vi "Create Tick Object.vi"(6 "Label Cluster In":T2, 8 "error in (no error)":errorcluster, 9 "Actual Range In":T1, 10 "3D Plot.lvclass in":refnum<class "3D Plot.lvclass">, 11 "Axis Object In":refnum<vi>) -> (0 "error out":errorcluster, 1 "Actual Range Out":T1, 2 "3D Plot.lvclass out":refnum<class "3D Plot.lvclass">, 3 "Axis Object Out":refnum<vi>, 4 "Label Cluster Out":T2)   [LabVIEW 2020, in "3D Plot.lvclass"]
uses:
  <vilib>/Math Plots/3D Math Plots/3D Plot/3D Plot/3D Plot.lvclass
  <vilib>/Math Plots/3D Math Plots/3D Plot/3D Plot/Typedef/Tick Array Cluster.ctl
  <vilib>/Math Plots/3D Math Plots/3D Plot/3D Plot/Typedef/Tick Array.ctl
  <vilib>/Math Plots/3D Math Plots/3D Plot/3D Plot/Typedef/Range Clusters.ctl
  <vilib>/Math Plots/3D Math Plots/3D Plot/3D Plot/3D Plot.lvclass/3D Plot.ctl
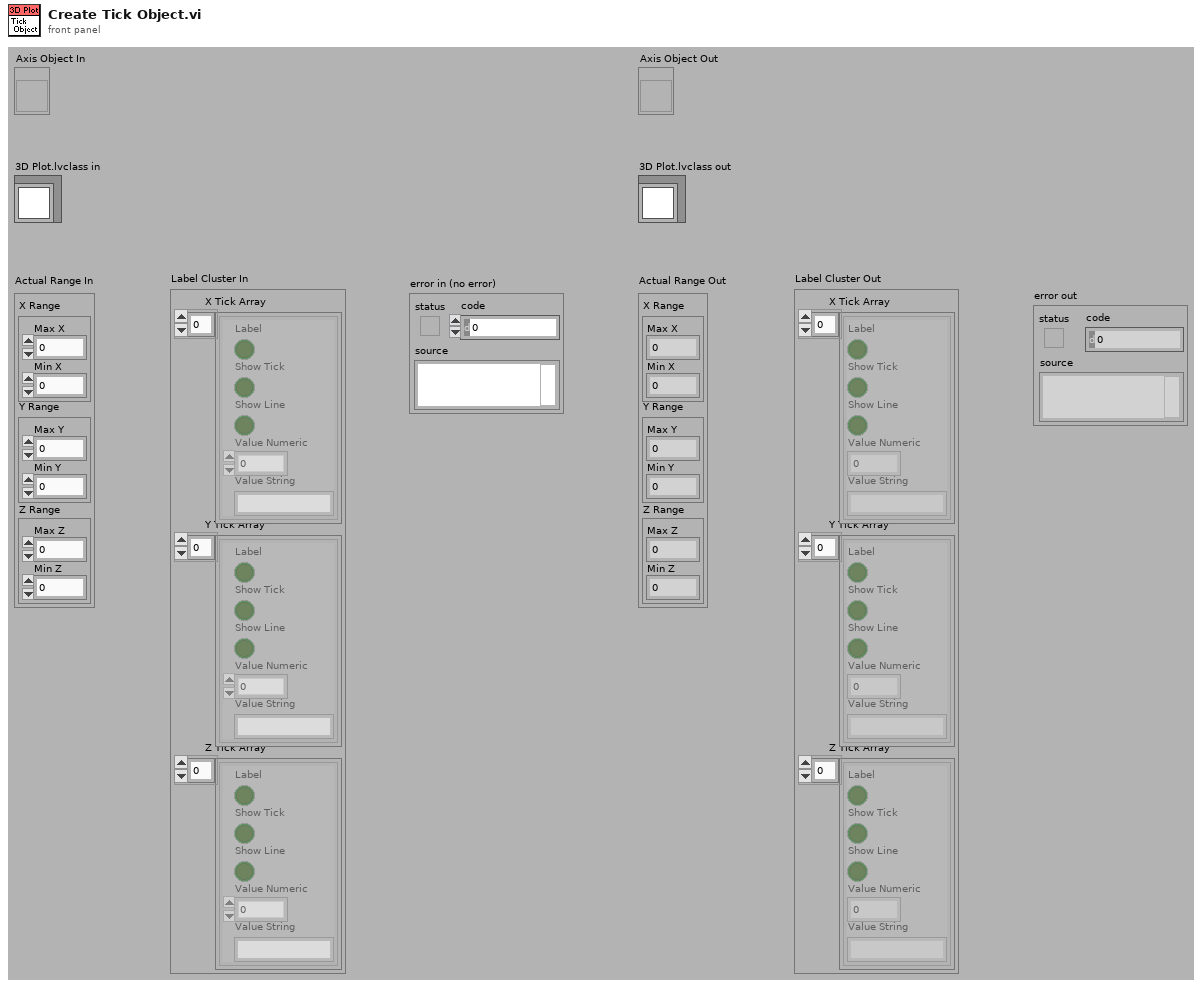
[diagram p1: front panel]
types:
  T1 = typedef "3D Plot.lvclass/Range Clusters.ctl" = cluster{"X Range":cluster{"Max X":sgl, "Min X":sgl}, "Y Range":cluster{"Max Y":sgl, "Min Y":sgl}, "Z Range":cluster{"Max Z":sgl, "Min Z":sgl}}
  T2 = typedef "3D Plot.lvclass/Tick Array Cluster.ctl" = cluster{"X Tick Array":T3, "Y Tick Array":T3, "Z Tick Array":T3}
  T3 = typedef "3D Plot.lvclass/Tick Array.ctl" = cluster{"Label":bool, "Show Tick":bool, "Show Line":bool, "Value Numeric":sgl, "Value String":string}[]
  T4 = cluster{"Draw Grid Plane X-Y":bool, "Draw Grid Plane Y-Z":bool, "Draw Grid Plane X-Z":bool}
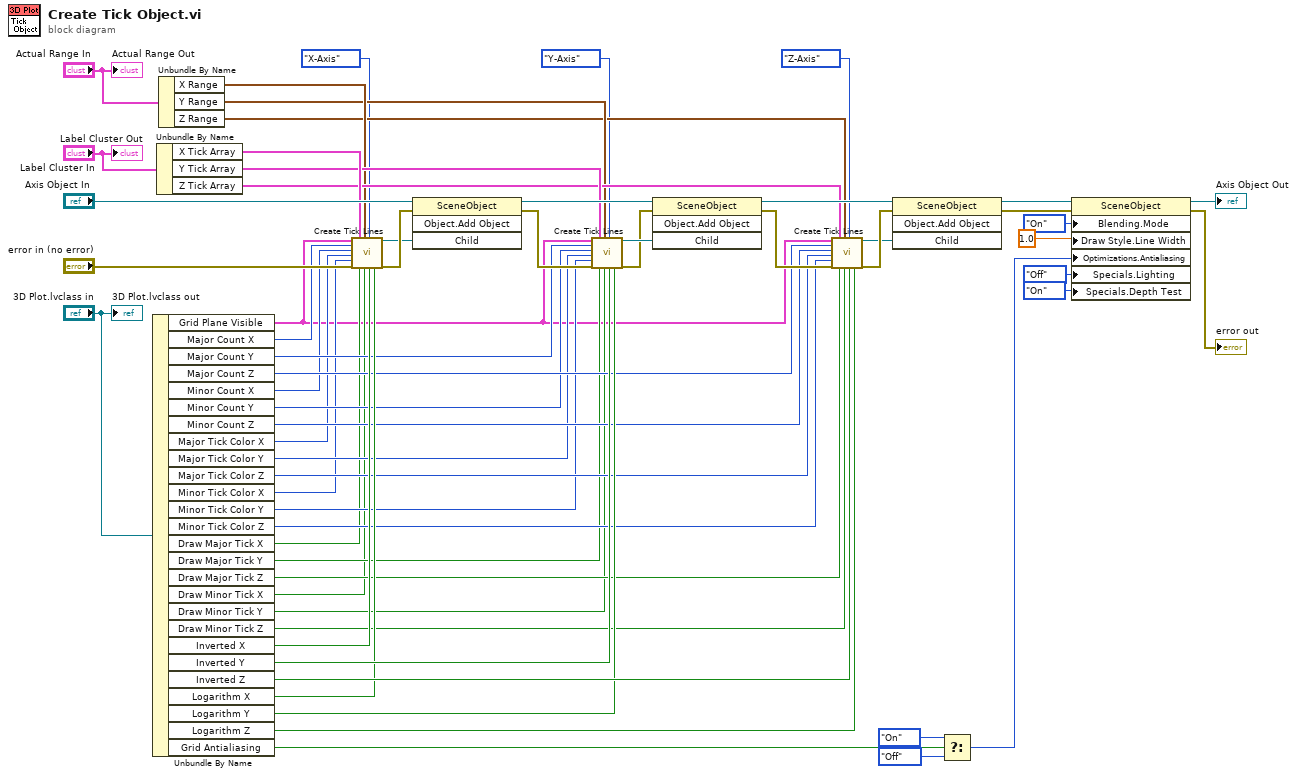
[diagram p0: block diagram]
diagram:
  n1 = Unbundle By Name("3D Plot.lvclass in") -> ("Grid Plane Visible"=w4:T4, "Major Count X"=w15:u16, "Major Count Y"=w38:u16, "Major Count Z"=w37:u16, "Minor Count X"=w36:u16, "Minor Count Y"=w35:u16, "Minor Count Z"=w34:u16, "Major Tick Color X"=w33:u32, "Major Tick Color Y"=w32:u32, "Major Tick Color Z"=w31:u32, "Minor Tick Color X"=w30:u32, "Minor Tick Color Y"=w29:u32, "Minor Tick Color Z"=w28:u32, "Draw Major Tick X"=w27:bool, "Draw Major Tick Y"=w26:bool, "Draw Major Tick Z"=w25:bool, "Draw Minor Tick X"=w24:bool, "Draw Minor Tick Y"=w23:bool, "Draw Minor Tick Z"=w22:bool, "Inverted X"=w46:bool, "Inverted Y"=w45:bool, "Inverted Z"=w44:bool, "Logarithm X"=w41:bool, "Logarithm Y"=w40:bool, "Logarithm Z"=w39:bool, "Grid Antialiasing"=w5:bool)
  n2 = Unbundle By Name("Label Cluster In") -> ("X Tick Array"=w52:T3, "Y Tick Array"=w51:T3, "Z Tick Array"=w50:T3)
  n3 = Unbundle By Name("Actual Range In") -> ("X Range"=w49:cluster{"Max X":sgl, "Min X":sgl}, "Y Range"=w48:cluster{"Max Y":sgl, "Min Y":sgl}, "Z Range"=w47:cluster{"Max Z":sgl, "Min Z":sgl})
  n4 = call <vilib>:"Create Tick Lines.vi"("Grid Plane Visible"=w4, "Major Ticks"=w15, "Minor Ticks"=w36, "Major Color"=w33, "Minor Color"=w30, "error in (no error)"="error in (no error)", "Tick Cluster Array"=w52, "Draw Major"=w27, "Range"=w49, "Draw Minor"=w24, "Axis"=enum16{"X-Axis", "Y-Axis", "Z-Axis"}."X-Axis", "Inverted?"=w46, "Logarithm?"=w41) -> ("Axis Tick Object Out"=w18:refnum<vi>, "error out"=w19:errorcluster)  [unwired: 1 in, 4 out]
  n5 = invoke class="SceneObject" method="Object.Add Object"(reference="Axis Object In", error in=w19, "Child"=w18) -> (reference out=w54:refnum<vi>, error out=w43:errorcluster)  [unwired: 1 in, 2 out]
  n6 = call <vilib>:"Create Tick Lines.vi"("Grid Plane Visible"=w4, "Major Ticks"=w38, "Minor Ticks"=w35, "Major Color"=w32, "Minor Color"=w29, "error in (no error)"=w43, "Tick Cluster Array"=w51, "Draw Major"=w26, "Range"=w48, "Draw Minor"=w23, "Axis"=enum16{"X-Axis", "Y-Axis", "Z-Axis"}."Y-Axis", "Inverted?"=w45, "Logarithm?"=w40) -> ("Axis Tick Object Out"=w21:refnum<vi>, "error out"=w20:errorcluster)  [unwired: 1 in, 4 out]
  n7 = invoke class="SceneObject" method="Object.Add Object"(reference=w54, error in=w20, "Child"=w21) -> (reference out=w53:refnum<vi>, error out=w42:errorcluster)  [unwired: 1 in, 2 out]
  n8 = call <vilib>:"Create Tick Lines.vi"("Grid Plane Visible"=w4, "Major Ticks"=w37, "Minor Ticks"=w34, "Major Color"=w31, "Minor Color"=w28, "error in (no error)"=w42, "Tick Cluster Array"=w50, "Draw Major"=w25, "Range"=w47, "Draw Minor"=w22, "Axis"=enum16{"X-Axis", "Y-Axis", "Z-Axis"}."Z-Axis", "Inverted?"=w44, "Logarithm?"=w39) -> ("Axis Tick Object Out"=w16:refnum<vi>, "error out"=w17:errorcluster)  [unwired: 1 in, 4 out]
  n9 = invoke class="SceneObject" method="Object.Add Object"(reference=w53, error in=w17, "Child"=w16) -> (reference out=w7:refnum<vi>, error out=w6:errorcluster)  [unwired: 1 in, 2 out]
  n10 = Select(t=enum16{"Inherit Value", "Off", "On"}."On" ("Optimizations:Antialiasing"), s=w5, f=enum16{"Inherit Value", "Off", "On"}."Off" ("Optimizations:Antialiasing")) -> (s? t:f=w8:enum16{"Inherit Value", "Off", "On"})
  n11 = property class="SceneObject"(reference=w7, error in=w6, "Blending.Mode"=enum16{"Inherit Value", "Off", "On"}."On" ("Specials:Lighting"), "Draw Style.Line Width"=sgl 1.0 ("Draw Style:Line Width"), "Optimizations.Antialiasing"=w8, "Specials.Lighting"=enum16{"Inherit Value", "Off", "On"}."Off" ("Blending:Mode"), "Specials.Depth Test"=enum16{"Inherit Value", "Off", "On"}."On" ("Specials:Depth Test")) -> (reference out=→"Axis Object Out":refnum<vi>, error out=→"error out":errorcluster)
  "Label Cluster Out" <- "Label Cluster In"
  "3D Plot.lvclass out" <- "3D Plot.lvclass in"
  "Actual Range Out" <- "Actual Range In"
